vi "HART_StartChar.vi"(10 "Message type":enum16{"Master to Slave", "Slave to Master"}(ring), 11 "Address type":enum16{"Short frame", "Long frame"}(ring)=enum."Long frame") -> (2 "start character":u8=130 format="%.0x")   [LabVIEW 2016]
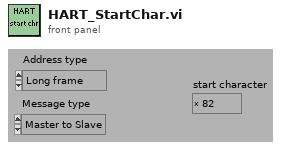
[diagram p1: front panel]
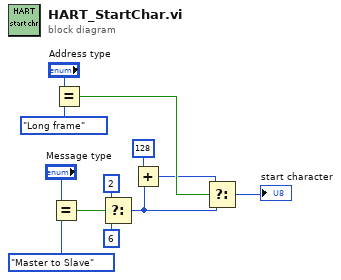
[diagram p0: block diagram]
diagram:
  n1 = Equal?(x="Message type", y=enum16{"Master to Slave", "Slave to Master"}."Master to Slave" ("Message type")) -> (x = y?=w10:bool)
  n2 = Equal?(x="Address type", y=enum16{"Short frame", "Long frame"}."Long frame" ("Address type")) -> (x = y?=w4:bool)
  n3 = Select(t=2, s=w10, f=6) -> (s? t:f=w2:i32)
  n4 = Add(x=128, y=w2) -> (x+y=w3:i32)
  n5 = Select(t=w3, s=w4, f=w2) -> (s? t:f=→"start character":i32)
